vi "Global compensazione attriti.vi"() -> ()   [LabVIEW 2019]
panel:
  in  "compensazione attriti":T1
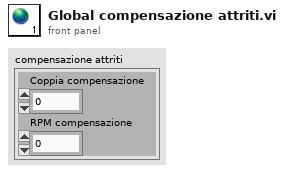
[diagram p1: front panel]
types:
  T1 = cluster{"Coppia compensazione":dbl, "RPM compensazione":dbl}
diagram:
